vi "Klinger SetAxisParams.vi"(0 "Axe":u8(ring) items=["W", "X", "Y", "Z"], 1 "TypeMouv":i32(ring) caption="Type de mouvement" items=["Linéaire", "Rotation"], 2 "Nom de l'axe":string, 5 "Type":i32(ring) caption="Type de moteur" items=["UE30", "UE72"], 7 "FactConv":dbl=0.01 caption="Facteur de\nConversion\n(m/pas ou °/pas)" format="%#_7g", 9 "CorrParams":T1={"CorrActive"=FALSE, "ErreurLim"=0.1, "NbrEssais"=3} caption="Paramètres de correction de position" {"NbrEssais" min=1 max=5 step=1; "ErreurLim" min=0.0 max=10.0 step=0.1 format="%#.1f"}, 11 "error in":errorcluster, 12 "Encodeur":bool caption="Possède un\nEncodeur", 13 "MiseàZéro":bool caption="Possède un\nInterrupteur d'origine") -> (15 "error out":errorcluster)   [LabVIEW 2010]
doc: "Ce Vi enregistre les paramètres des différents axes dans un fichier .ini"
uses:
  <vilib>/Utility/config.llb/Write Key (I32).vi
  <vilib>/Utility/config.llb/Write Key (Boolean).vi
  <vilib>/Utility/config.llb/Write Key (Double).vi
  <vilib>/Utility/config.llb/Write Key (String).vi
  <vilib>/Utility/config.llb/NI_LVConfig.lvlib
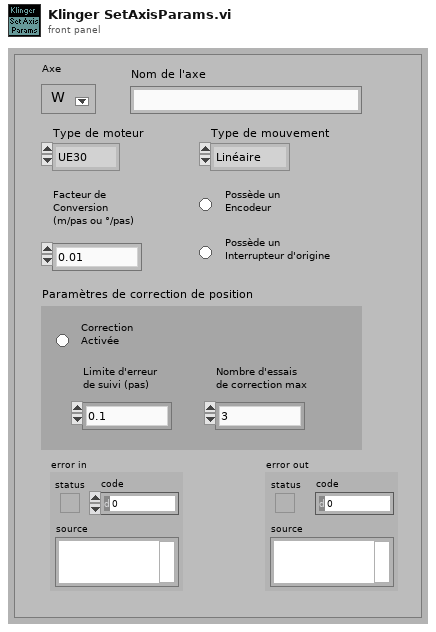
[diagram p1: front panel]
types:
  T1 = cluster{"CorrActive":bool, "ErreurLim":dbl, "NbrEssais":i32}
  T2 = typedef "NI_LVConfig.lvlib/Config Data RefNum.ctl" = refnum<k1>
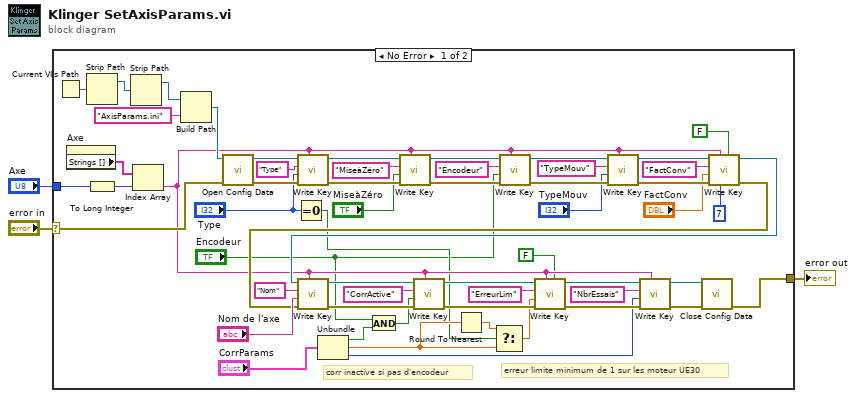
[diagram p0: block diagram]
diagram:
  n1 = case shown="No Error" "error in" {
    selector: "error in" -> [w55 w61]
    tunnel: "Axe" -> [w54 _]
    tunnel: [w16 w61] -> w2
    frame No Error {
      # "erreur limite minimum de 1 sur les moteur UE30"
      # "corr inactive si pas d'encodeur"
      n2 = Current VI's Path() -> (path=w60:path)
      n3 = property on="Axe" class="Ring (strict)"() -> ("Strings []"=w52:string[])  [unwired: 2 in, 2 out]
      n4 = Strip Path(path=w60) -> (stripped path=w59:path)  [unwired: 1 out]
      n5 = To Long Integer(number=w54) -> (32bit integer=w53:i32)
      n6 = Strip Path(path=w59) -> (stripped path=w58:path)  [unwired: 1 out]
      n7 = Index Array(array=w52, index=w53) -> (element=w15:string)
      n8 = Build Path(base path=w58, name or relative path="AxisParams.ini") -> (appended path=w56:path)
      n9 = call <vilib>:"Open Config Data.vi"("error in (no error)"=w55, "configuration file path"=w56) -> ("error out"=w42:errorcluster, "refnum"=w43:T2)  [unwired: 7 in, 1 out]
      n10 = Equal To 0?(x="Type") -> (x = 0?=w10:bool)
      n11 = call-poly <vilib>:"Write Key.vi"("section"=w15, "error in (no error)"=w42, "value"="Type", "key"="Type", "refnum"=w43) -> ("error out"=w39:errorcluster, "refnum out"=w41:T2)  [unwired: 4 in, 1 out]
      n12 = Unbundle("CorrParams") -> ("CorrActive"=w9:bool, "ErreurLim"=w12:dbl, "NbrEssais"=w19:i32)
      n13 = And(x="Encodeur", y=w9) -> (x .and. y?=w7:bool)
      n14 = call-poly <vilib>:"Write Key.vi"("section"=w15, "error in (no error)"=w39, "value"="MiseàZéro", "key"="MiseàZéro", "refnum"=w41) -> ("error out"=w37:errorcluster, "refnum out"=w32:T2)  [unwired: 4 in, 1 out]
      n15 = Round To Nearest(number=w12) -> (nearest integer value=w13:dbl)
      n16 = Select(t=w13, s=w10, f=w12) -> (s? t:f=w11:dbl)
      n17 = call-poly <vilib>:"Write Key.vi"("section"=w15, "error in (no error)"=w37, "value"="Encodeur", "key"="Encodeur", "refnum"=w32) -> ("error out"=w36:errorcluster, "refnum out"=w33:T2)  [unwired: 4 in, 1 out]
      n18 = call-poly <vilib>:"Write Key.vi"("section"=w15, "error in (no error)"=w36, "value"="TypeMouv", "key"="TypeMouv", "refnum"=w33) -> ("error out"=w35:errorcluster, "refnum out"=w34:T2)  [unwired: 4 in, 1 out]
      n19 = call-poly <vilib>:"Write Key.vi"("use system decimal point (T)"=FALSE, "precision (6)"=i16 7, "section"=w15, "error in (no error)"=w35, "value"="FactConv", "key"="FactConv", "refnum"=w34) -> ("error out"=w26:errorcluster, "refnum out"=w27:T2)  [unwired: 2 in, 1 out]
      n20 = call-poly <vilib>:"Write Key.vi"("section"=w15, "error in (no error)"=w26, "value"="Nom de l'axe", "key"="Nom", "refnum"=w27) -> ("error out"=w24:errorcluster, "refnum out"=w25:T2)  [unwired: 4 in, 1 out]
      n21 = call-poly <vilib>:"Write Key.vi"("section"=w15, "error in (no error)"=w24, "value"=w7, "key"="CorrActive", "refnum"=w25) -> ("error out"=w22:errorcluster, "refnum out"=w23:T2)  [unwired: 4 in, 1 out]
      n22 = call-poly <vilib>:"Write Key.vi"("use system decimal point (T)"=FALSE, "section"=w15, "error in (no error)"=w22, "value"=w11, "key"="ErreurLim", "refnum"=w23) -> ("error out"=w20:errorcluster, "refnum out"=w21:T2)  [unwired: 3 in, 1 out]
      n23 = call-poly <vilib>:"Write Key.vi"("section"=w15, "error in (no error)"=w20, "value"=w19, "key"="NbrEssais", "refnum"=w21) -> ("error out"=w17:errorcluster, "refnum out"=w18:T2)  [unwired: 4 in, 1 out]
      n24 = call <vilib>:"Close Config Data.vi"("error in (no error)"=w17, "refnum"=w18) -> ("error out"=w16:errorcluster)  [unwired: 8 in, 1 out]
    }
    frame Error {
    }
  }
  "error out" <- w2
